vi "Drive 4.vi"(6 "Rotation":dbl, 7 "Gyro Angle":dbl, 8 "error in (no error)":errorcluster, 9 "Y":dbl, 10 "X":dbl, 11 "RobotDriveDevRef 2":T1={"DevStatus"={"status"=FALSE, "code"=0, "source"=""}, "Motors[]"=[], "Square Inputs"=FALSE, "Max Output"=1.0, "Isochronous"=FALSE}) -> (0 "error out":errorcluster, 2 "Motor Values":dbl[](array[numeric]), 3 "RobotDriveDevRef":T1={"DevStatus"={"status"=FALSE, "code"=0, "source"=""}, "Motors[]"=[], "Square Inputs"=FALSE, "Max Output"=1.0, "Isochronous"=FALSE})   [LabVIEW 2013]
uses:
  <vilib>/Rock Robotics/WPI/RobotDrive/WPI_RobotDriveDevRef.ctl
  <vilib>/Rock Robotics/WPI/MotorControl/WPI_MotorControlDeviceRef.ctl
  <vilib>/Rock Robotics/SystemInterfaces/Typedef/FPGA_TypedefDigitalModule.ctl
  <vilib>/Rock Robotics/SystemInterfaces/DIO/FPGA_DIOPWMChannel.ctl
  <vilib>/Rock Robotics/WPI/PWM/WPI_PWMDeadband.ctl
  <vilib>/Rock Robotics/WPI/CAN/Jaguar/SubVIs/WPI_CANJaguar_ControlMode.ctl
  <vilib>/Rock Robotics/WPI/PWM/WPI_PWMTransform_ConPane.ctl
  <vilib>/Rock Robotics/SystemInterfaces/NetworkCommunication/NetComm_UsageReport_ResourceType.ctl
  <vilib>/Rock Robotics/WPI/RobotDrive/WPI_RobotDriveMotorSelectorEnum.ctl
  <vilib>/Rock Robotics/WPI/RobotDrive/WPI_RobotDriveSafetyCheck.vi
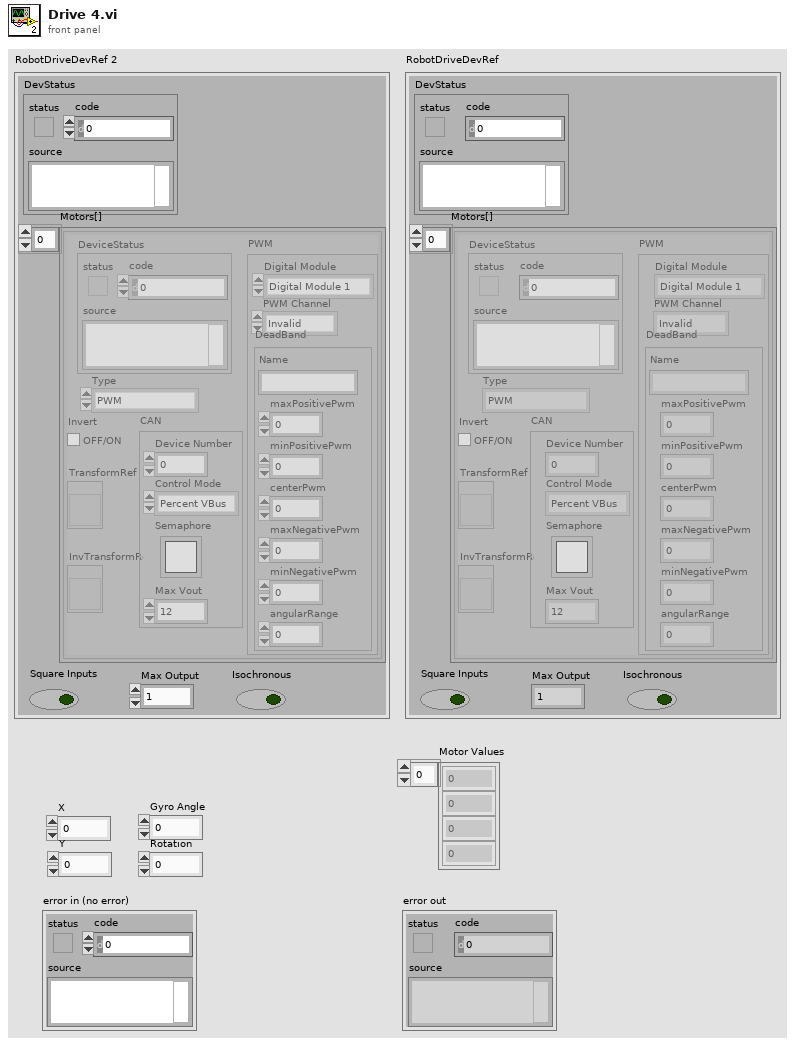
[diagram p1: front panel]
types:
  T1 = typedef "WPI_RobotDriveDevRef.ctl" = cluster{"DevStatus":errorcluster, "Motors[]":T2[], "Square Inputs":bool, "Max Output":dbl, "Isochronous":bool}
  T2 = typedef "WPI_MotorControlDeviceRef.ctl" = cluster{"DeviceStatus":errorcluster, "Type":enum16{"PWM", "CAN"}, "PWM":cluster{"Digital Module":T3, "PWM Channel":T4, "DeadBand":T5}, "CAN":cluster{"Device Number":u8, "Control Mode":T6, "Semaphore":T7, "Max Vout":dbl}, "Invert":bool, "TransformRef":T8, "InvTransformRef":T8}
  T3 = typedef "FPGA_TypedefDigitalModule.ctl" = enum16{"Digital Module 1", "Digital Module 2"}
  T4 = typedef "FPGA_DIOPWMChannel.ctl" = enum8{"PWM 1", "PWM 2", "PWM 3", "PWM 4", "PWM 5", "PWM 6", "PWM 7", "PWM 8", "PWM 9", "PWM 10", "Invalid"}
  T5 = typedef "WPI_PWMDeadband.ctl" = cluster{"Name":string, "maxPositivePwm":i32, "minPositivePwm":i32, "centerPwm":i32, "maxNegativePwm":i32, "minNegativePwm":i32, "angularRange":u16}
  T6 = typedef "WPI_CANJaguar_ControlMode.ctl" = enum8{"Percent VBus", "Current", "Speed", "Position", "Voltage"}
  T7 = typedef "Semaphore RefNum" = refnum<k1>
  T8 = typedef "WPI_PWMTransform_ConPane.ctl" = refnum<vi>
  T9 = typedef "NetComm_UsageReport_ResourceType.ctl" = enum8{"Controller", "Module", "Language", "CANPlugin", "Accelerometer", "ADXL345", "AnalogChannel", "AnalogTrigger", "AnalogTriggerOutput", "CANJaguar", "Compressor", "Counter", "Dashboard", "DigitalInput", "DigitalOutput", "DriverStationCIO", "DriverStationEIO", "DriverStationLCD", "Encoder", "GearTooth", "Gyro", "I2C", "Framework", "Jaguar", "Joystick", "Kinect", "KinectStick", "PIDController", "Preferences", "PWM", "Relay", "RobotDrive", "SerialPort", "Servo", "Solenoid", "SPI", "Task", "Ultrasonic", "Victor", "Button", "Command", "AxisCamera", "PCVideoServer", "SmartDashboard", "Talon", "HiTechnicColorSensor", "HiTechnicAccel", "HiTechnicCompass", "SRF08"}
  T10 = typedef "WPI_RobotDriveMotorSelectorEnum.ctl" = enum16{"Rear Left Motor", "Rear Right Motor", "Front Left Motor", "Front Right Motor"}
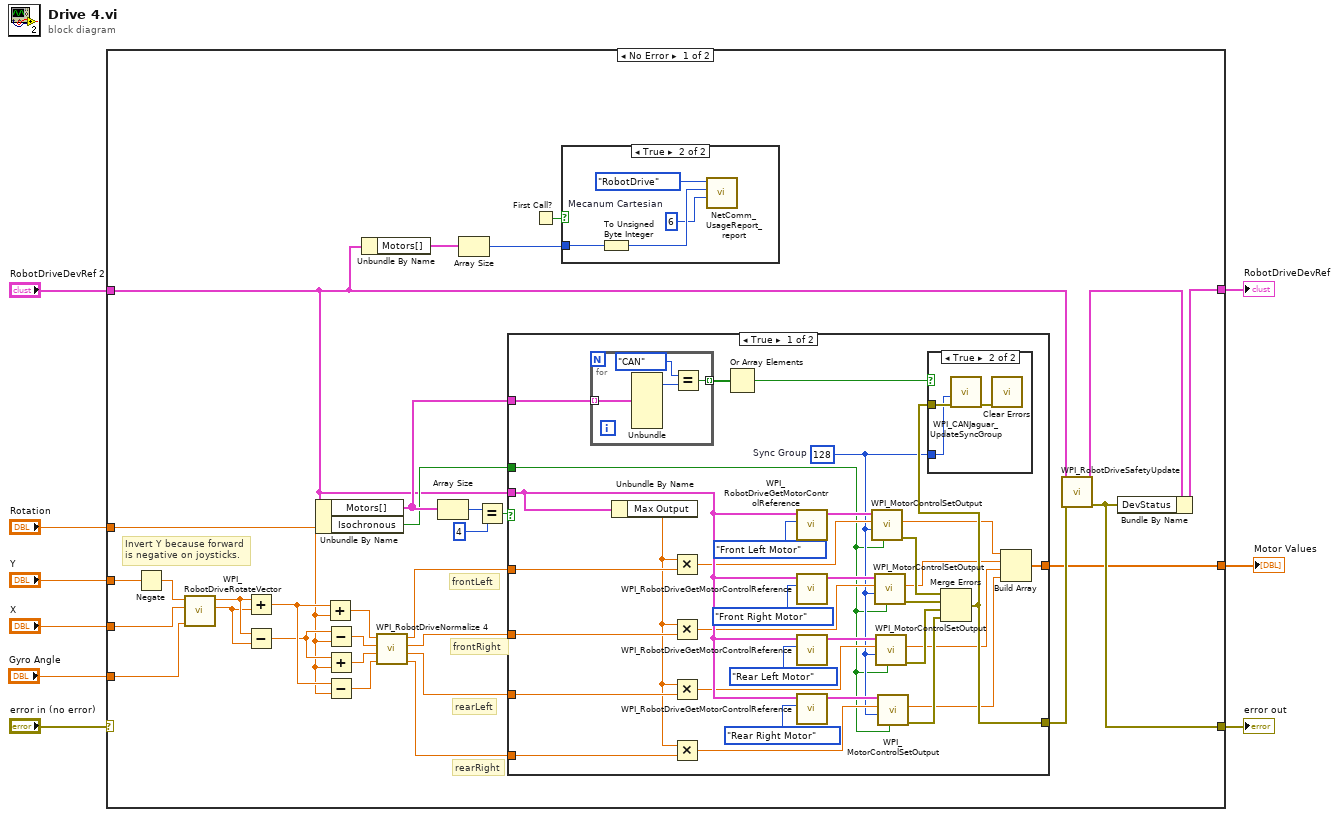
[diagram p0: block diagram]
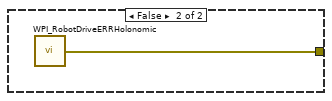
[diagram p4: hidden frame]
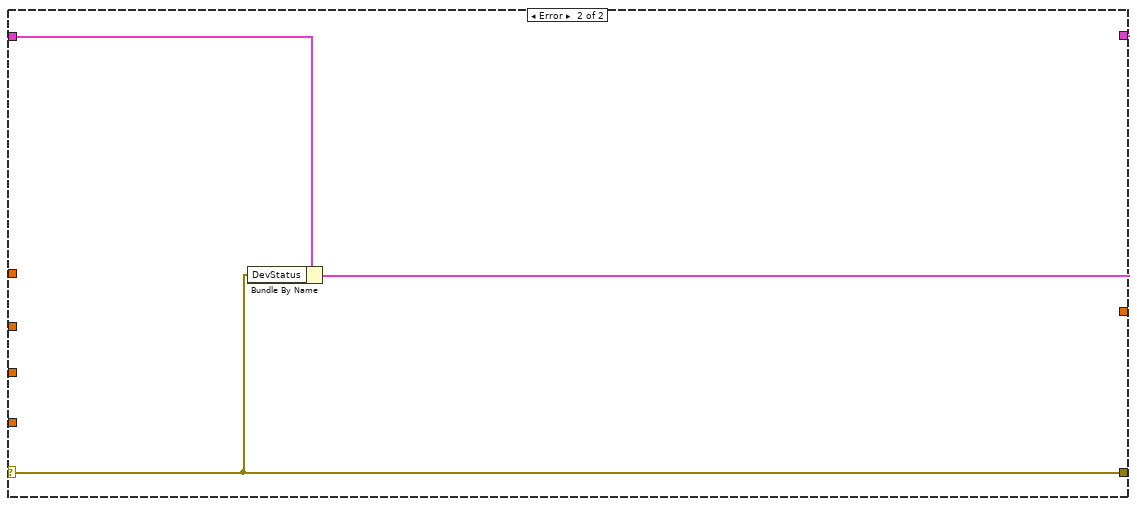
[diagram p5: hidden frame]
diagram:
  n1 = case shown="No Error" "error in (no error)" {
    selector: "error in (no error)" -> [_ w86]
    tunnel: "Y" -> [w22 _]
    tunnel: "X" -> [w27 _]
    tunnel: "RobotDriveDevRef 2" -> [w11 w88]
    tunnel: [w37 w87] -> w5
    tunnel: [w17 w86] -> w4
    tunnel: "Rotation" -> [w28 _]
    tunnel: "Gyro Angle" -> [w21 _]
    tunnel: [w10 _] -> w1
    frame No Error {
      # "Invert Y because forward is negative on joysticks."
      # "rearLeft"
      # "frontRight"
      # "rearRight"
      # "frontLeft"
      n2 = Negate(x=w22) -> (-x=w20:dbl)
      n3 = call <vilib>:"WPI_RobotDriveRotateVector.vi"("Angle"=w21, "X"=w27, "Y"=w20) -> ("X'"=w35:dbl, "Y'"=w36:dbl)  [unwired: 7 out]
      n4 = Add(x=w36, y=w35) -> (x+y=w33:dbl)
      n5 = Subtract(x=w36, y=w35) -> (x-y=w31:dbl)
      n6 = Unbundle By Name(w11) -> ("Motors[]"=w16:T2[], "Isochronous"=w15:bool)
      n7 = Add(x=w33, y=w28) -> (x+y=w29:dbl)
      n8 = Subtract(x=w31, y=w28) -> (x-y=w30:dbl)
      n9 = Add(x=w31, y=w28) -> (x+y=w32:dbl)
      n10 = Subtract(x=w33, y=w28) -> (x-y=w34:dbl)
      n11 = Unbundle By Name(w11) -> ("Motors[]"=w13:T2[])
      n12 = call <vilib>:"WPI_RobotDriveNormalize 4.vi"("D"=w34, "C"=w32, "B"=w30, "A"=w29) -> ("D'"=w24:dbl, "C'"=w23:dbl, "B'"=w25:dbl, "A'"=w26:dbl)
      n13 = Array Size(array=w16) -> (size(s)=w40:i32)
      n14 = Array Size(array=w13) -> (size(s)=w12:i32)
      n15 = Equal?(x=w40, y=4) -> (x = y?=w38:bool)
      n16 = case shown="True" w38 {
        tunnel: w26 -> [w77 _]
        tunnel: w25 -> [w76 _]
        tunnel: w11 -> [w65 _]
        tunnel: [w52 w85] -> w19
        tunnel: w23 -> [w71 _]
        tunnel: w24 -> [w70 _]
        tunnel: w16 -> [w53 _]
        tunnel: w15 -> [w50 _]
        tunnel: [w48 _] -> w10
        frame True {
          w51 = u8 128  # Sync Group
          n17 = for {
            tunnel: w53 -> [w81] mode=indexing
            tunnel: [w78] -> w54 mode=indexing
            n18 = Unbundle(w81) -> ("Type"=w80:enum16{"PWM", "CAN"})  [unwired: 6 out]
            n19 = Equal?(x=enum16{"PWM", "CAN"}."CAN" ("Type"), y=w80) -> (x = y?=w78:bool)
          }
          n20 = Unbundle By Name(w65) -> ("Max Output"=w60:dbl)
          n21 = Multiply(x=w60, y=w77) -> (x*y=w64:dbl)
          n22 = Multiply(x=w60, y=w76) -> (x*y=w63:dbl)
          n23 = Multiply(x=w60, y=w71) -> (x*y=w62:dbl)
          n24 = Multiply(x=w60, y=w70) -> (x*y=w61:dbl)
          n25 = Or Array Elements(Boolean array=w54) -> (logical OR=w55:bool)
          n26 = call <vilib>:"WPI_RobotDriveGetMotorControlReference.vi"("MotorIndex"=WPI_RobotDriveMotorSelectorEnum."Front Left Motor", "RobotDriveDevRef"=w65) -> ("MotorControlDeviceRef"=w75:T2)  [unwired: 9 out]
          n27 = call <vilib>:"WPI_RobotDriveGetMotorControlReference.vi"("MotorIndex"=WPI_RobotDriveMotorSelectorEnum."Front Right Motor", "RobotDriveDevRef"=w65) -> ("MotorControlDeviceRef"=w73:T2)  [unwired: 9 out]
          n28 = call <vilib>:"WPI_RobotDriveGetMotorControlReference.vi"("MotorIndex"=WPI_RobotDriveMotorSelectorEnum."Rear Left Motor", "RobotDriveDevRef"=w65) -> ("MotorControlDeviceRef"=w74:T2)  [unwired: 9 out]
          n29 = call <vilib>:"WPI_RobotDriveGetMotorControlReference.vi"("MotorIndex"=WPI_RobotDriveMotorSelectorEnum."Rear Right Motor", "RobotDriveDevRef"=w65) -> ("MotorControlDeviceRef"=w72:T2)  [unwired: 9 out]
          n30 = call <vilib>:"WPI_MotorControlSetOutput.vi"("Isochronous"=w50, "Sync Group"=w51, "Output"=w64, "MotorControlDevRef"=w75) -> ("error out"=w56:errorcluster, "Motor Output"=w49:dbl)  [unwired: 1 in, 5 out]
          n31 = call <vilib>:"WPI_MotorControlSetOutput.vi"("Isochronous"=w50, "Sync Group"=w51, "Output"=w63, "MotorControlDevRef"=w73) -> ("error out"=w57:errorcluster, "Motor Output"=w47:dbl)  [unwired: 1 in, 5 out]
          n32 = call <vilib>:"WPI_MotorControlSetOutput.vi"("Isochronous"=w50, "Sync Group"=w51, "Output"=w62, "MotorControlDevRef"=w74) -> ("error out"=w58:errorcluster, "Motor Output"=w46:dbl)  [unwired: 1 in, 5 out]
          n33 = call <vilib>:"WPI_MotorControlSetOutput.vi"("Isochronous"=w50, "Sync Group"=w51, "Output"=w61, "MotorControlDevRef"=w72) -> ("error out"=w59:errorcluster, "Motor Output"=w45:dbl)  [unwired: 1 in, 5 out]
          n34 = Merge Errors(w56, w57, w58, w59) -> (w52:errorcluster)
          n35 = case shown="True" w55 {
            tunnel: w52 -> [_ w83]
            tunnel: w51 -> [_ w82]
            frame False {
            }
            frame True {
              n36 = call <vilib>:"WPI_CANJaguar_UpdateSyncGroup.vi"("error in (no error)"=w83, "Sync Group"=w82) -> ("error out"=w84:errorcluster)  [unwired: 9 out]
              n37 = call <vilib>:"Clear Errors.vi"("error in (no error)"=w84) -> ()  [unwired: 7 out]
            }
          }
          n38 = Build Array(w49, w47, w46, w45) -> (w48:dbl[])
        }
        frame False {
          n39 = call <vilib>:"WPI_RobotDriveERRHolonomic.vi"() -> ("error out"=w85:errorcluster)
        }
      }
      n40 = First Call?() -> (First Call?: T/F=w14:bool)
      n41 = case shown="True" w14 {
        tunnel: w12 -> [_ w43]
        frame False {
        }
        frame True {
          w41 = u8 6  # Mecanum Cartesian
          n42 = To Unsigned Byte Integer(number=w43) -> (unsigned 8bit integer=w42:u8)
          n43 = call <vilib>:"NetComm_UsageReport_report.vi"("Context"=w41, "Instance Number"=w42, "Resource Type"=NetComm_UsageReport_ResourceType."RobotDrive") -> ()  [unwired: 9 in]
        }
      }
      n44 = call <vilib>:"WPI_RobotDriveSafetyUpdate.vi"("error in (no error)"=w19, "RobotDriveDevRef"=w11) -> ("error out"=w17:errorcluster, "RobotDriveDevRef"=w18:T1)  [unwired: 8 out]
      n45 = Bundle By Name(cluster=w18, "DevStatus"=w17) -> (w37:T1)
    }
    frame Error {
      n46 = Bundle By Name(cluster=w88, "DevStatus"=w86) -> (w87:T1)
    }
  }
  "error out" <- w4
  "RobotDriveDevRef" <- w5
  "Motor Values" <- w1
